vi "UART_Read_Write.vi"(0 "Transmit":refnum<k21>="Port8/DIO0", 5 "Receive":refnum<k21>="Port8/DIOCTL", 7 "baud rate (9600)":u32=9600, 9 "data bits (8)":i32=8 min=5 max=8 step=1, 11 "parity (0:none)":enum16{"None", "Odd", "Even", "Mark", "Space"}(ring), 12 "stop bits (10: 1 bit)":u16(ring)=10 items=["1.0"=10, "1.5"=15, "2.0"=20], 13 "Invert Polarity?":bool) -> ()   [LabVIEW 2011]
uses:
  <vilib>/rvi/eio/common/nirviEmuTemplateMethod_errors.vi
  <vilib>/rvi/interface/RandomDataEmulation/nirviRandomDataFPGAFIFO.vi
  <vilib>/rvi/interface/RandomDataEmulation/niFpgaRandomDataHandleErrors.vi
  Instance           1 27Saved   LV FPGA Serial Read .vi
  Instance           2 27Saved   LV FPGA Serial Read .vi
  Instance           3 27Saved   LV FPGA Serial Read .vi
  Instance           6 27Saved   LV FPGA Serial Read .vi
  <vilib>/eio/EIOMethodNode/EIOMethodNode.xnode
  <vilib>/rvi/DataTransferAndStorage/Container/XNode/niFpgaContainer.xnode
  <vilib>/rvi/interface/RandomDataEmulation/nirviRandomDataFpgaReadWriteTemplate.vi
  <vilib>/eio/EIONode/EIONode.xnode
panel:
  out "Read: Transmission Error":bool
  in  "stop":bool
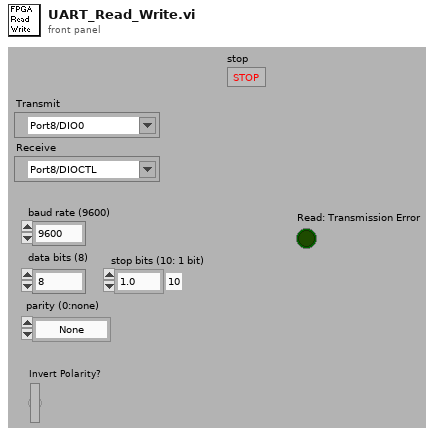
[diagram p1: front panel]
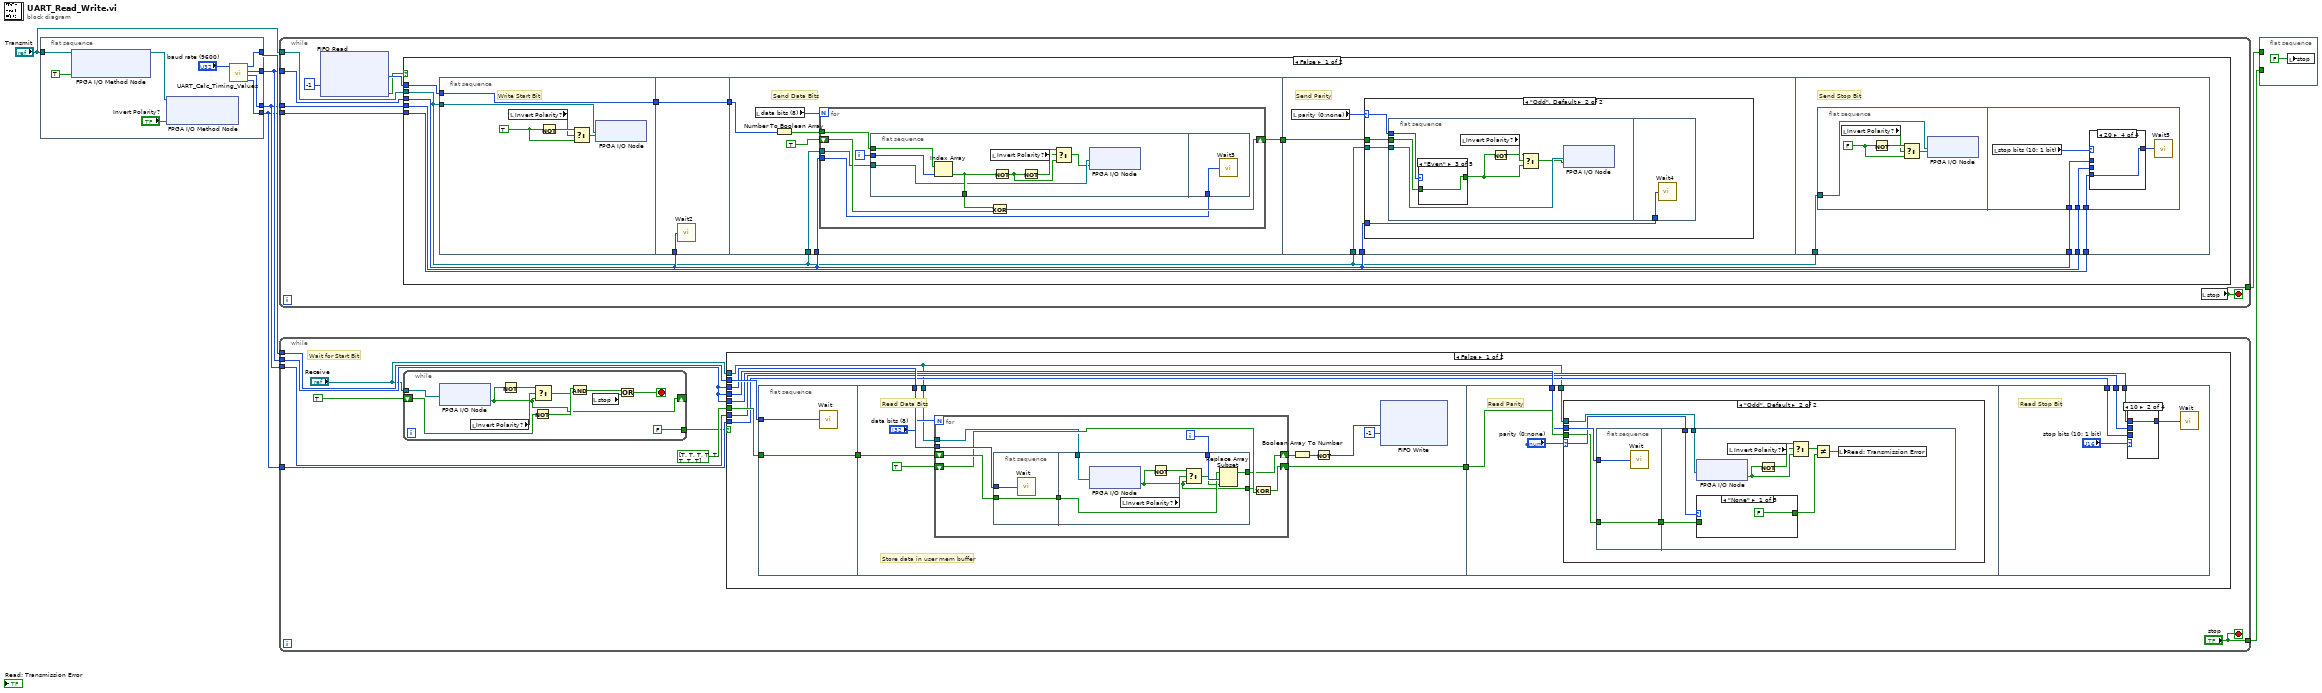
[diagram p0: block diagram]
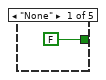
[diagram p3: hidden frame]
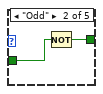
[diagram p4: hidden frame]
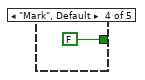
[diagram p5: hidden frame]
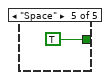
[diagram p6: hidden frame]
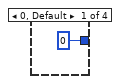
[diagram p7: hidden frame]
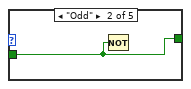
[diagram p12: hidden frame]
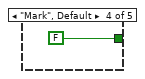
[diagram p14: hidden frame]
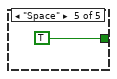
[diagram p15: hidden frame]
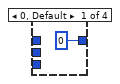
[diagram p16: hidden frame]
diagram:
  n1 = flat-sequence {
    tunnel: [w12] -> w6
    tunnel: [w15] -> w7
    tunnel: [w14] -> w5
    tunnel: [w13] -> w4
    tunnel: "Transmit" -> [w10]
    frame #0 {
      n2 = xnode "FPGA I/O Method Node"("FPGA I/O In"=w10, "Enable"=TRUE ("Digital Enable")) -> ("FPGA I/O Out"=w9:refnum<k21>)
      n3 = xnode "FPGA I/O Method Node"("FPGA I/O In"=w9, "Data"="Invert Polarity?") -> ()  [unwired: 1 out]
      n4 = call "UART_Calc_Timing_Values.vi"("baud rate (1000000)"="baud rate (9600)") -> ("Two Bit"=w13:u32, "One and Half Bit"=w14:u32, "One Bit"=w12:u32, "Half Bit"=w15:u32)  [unwired: 1 in, 2 out]
    }
  }
  n5 = while {
    tunnel: w4 -> [w24]
    tunnel: w5 -> [w23]
    tunnel: w6 -> [w22]
    tunnel: "Transmit" -> [w21]
    tunnel: [w17] -> w1
    stop <- w17 stop-if-true
    n6 = xnode ("FIFO Read")("Timeout"=-1) -> ("Element"=w20:u8, "Timed Out?"=w18:bool)  [unwired: 1 in, 1 out]
    n7 = case shown="False" w18 {
      tunnel: w24 -> [w29 _]
      tunnel: w23 -> [w28 _]
      tunnel: w22 -> [w27 _]
      tunnel: w21 -> [w26 _]
      tunnel: w20 -> [w25 _]
      frame False {
        n8 = flat-sequence {
          tunnel: w26 -> [w38]
          tunnel: w25 -> [w33]
          tunnel: [w33] -> w32
          tunnel: w27 -> [w40]
          tunnel: [w39] -> w31
          tunnel: w32 -> [w39]
          tunnel: w27 -> [w47]
          tunnel: [w45] -> w30
          tunnel: w26 -> [w42]
          tunnel: w31 -> [w41]
          tunnel: w27 -> [w66]
          tunnel: w30 -> [w67]
          tunnel: w26 -> [w64]
          tunnel: w27 -> [w89]
          tunnel: w28 -> [w88]
          tunnel: w29 -> [w87]
          tunnel: w26 -> [w86]
          frame #0 {
            w36 = TRUE
            # "Write Start Bit"
            n9 = local read "Invert Polarity?"() -> (w35:bool)
            n10 = Not(x=w36) -> (.not. x?=w37:bool)
            n11 = Select(t=w37, s=w35, f=w36) -> (s? t:f=w34:bool)
            n12 = xnode "FPGA I/O Node"("I/O Item"=w34, "FPGA I/O In"=w38) -> ()  [unwired: 1 out]
          }
          frame #1 {
            n13 = call "Wait2"("Count(Ticks)"=w40) -> ()  [unwired: 1 out]
          }
          frame #2 {
            # "Send Data Bits"
            n14 = local read "data bits (8)"() -> (w43:i32)
            n15 = Number To Boolean Array(number=w41) -> (Boolean array=w44:bool[])
            n16 = for {
              N: w43 -> [_]
              tunnel: w47 -> [w51]
              shift-right: [w54] -> w45
              shift-left: TRUE -> [w53]
              tunnel: w44 -> [w50]
              tunnel: w42 -> [w48]
              i -> [w52]
              n17 = flat-sequence {
                tunnel: w52 -> [w62]
                tunnel: w50 -> [w61]
                tunnel: [w60] -> w49
                tunnel: w48 -> [w59]
                tunnel: w51 -> [w63]
                frame #0 {
                  n18 = Index Array(array=w61, index=w62) -> (element=w60:bool)
                  n19 = local read "Invert Polarity?"() -> (w56:bool)
                  n20 = Not(x=w60) -> (.not. x?=w57:bool)
                  n21 = Not(x=w57) -> (.not. x?=w58:bool)
                  n22 = Select(t=w58, s=w56, f=w57) -> (s? t:f=w55:bool)
                  n23 = xnode "FPGA I/O Node"("I/O Item"=w55, "FPGA I/O In"=w59) -> ()  [unwired: 1 out]
                }
                frame #1 {
                  n24 = call "Wait3"("Count(Ticks)"=w63) -> ()  [unwired: 1 out]
                }
              }
              n25 = Exclusive Or(1:w53, 2:w49) -> (0:w54:bool)
            }
          }
          frame #3 {
            # "Send Parity"
            n26 = local read "parity (0:none)"() -> (w65:enum16{"None", "Odd", "Even", "Mark", "Space"})
            n27 = case shown="\"Odd\", Default" w65 {
              selector: w65 -> [_ w71]
              tunnel: w67 -> [_ w70]
              tunnel: w66 -> [_ w69]
              tunnel: w64 -> [_ w68]
              frame "None" {
              }
              frame "Odd", Default {
                n28 = flat-sequence {
                  tunnel: w70 -> [w77]
                  tunnel: w71 -> [w78]
                  tunnel: w68 -> [w76]
                  tunnel: w69 -> [w85]
                  frame #0 {
                    n29 = case shown="\"Even\"" w78 {
                      tunnel: w77 -> [_ w81 w82 _ _]
                      tunnel: [FALSE ("y") w80 w82 FALSE ("y") TRUE ("y")] -> w73
                      frame "None" {
                      }
                      frame "Odd" {
                        n30 = Not(x=w81) -> (.not. x?=w80:bool)
                      }
                      frame "Even" {
                      }
                      frame "Mark", Default {
                      }
                      frame "Space" {
                      }
                    }
                    n31 = local read "Invert Polarity?"() -> (w75:bool)
                    n32 = Not(x=w73) -> (.not. x?=w74:bool)
                    n33 = Select(t=w74, s=w75, f=w73) -> (s? t:f=w72:bool)
                    n34 = xnode "FPGA I/O Node"("I/O Item"=w72, "FPGA I/O In"=w76) -> ()  [unwired: 1 out]
                  }
                  frame #1 {
                    n35 = call "Wait4"("Count(Ticks)"=w85) -> ()  [unwired: 1 out]
                  }
                }
              }
            }
          }
          frame #4 {
            # "Send Stop Bit"
            n36 = flat-sequence {
              tunnel: w86 -> [w94]
              tunnel: w89 -> [w99]
              tunnel: w88 -> [w98]
              tunnel: w87 -> [w97]
              frame #0 {
                w92 = FALSE
                n37 = local read "Invert Polarity?"() -> (w91:bool)
                n38 = Not(x=w92) -> (.not. x?=w93:bool)
                n39 = Select(t=w93, s=w91, f=w92) -> (s? t:f=w90:bool)
                n40 = xnode "FPGA I/O Node"("I/O Item"=w90, "FPGA I/O In"=w94) -> ()  [unwired: 1 out]
              }
              frame #1 {
                n41 = local read "stop bits (10: 1 bit)"() -> (w95:u16)
                n42 = case shown="20" w95 {
                  tunnel: w99 -> [_ w101 _ _]
                  tunnel: w98 -> [_ _ w102 _]
                  tunnel: w97 -> [_ _ _ w103]
                  tunnel: [u32 0 ("One Bit") w101 w102 w103] -> w96
                  frame 0, Default {
                  }
                  frame 10 {
                  }
                  frame 15 {
                  }
                  frame 20 {
                  }
                }
                n43 = call "Wait5"("Count(Ticks)"=w96) -> ()  [unwired: 1 out]
              }
            }
          }
        }
      }
      frame True {
      }
    }
    n44 = local read "stop"() -> (w17:bool)
  }
  n45 = while {
    tunnel: w4 -> [w111]
    tunnel: w5 -> [w110]
    tunnel: w6 -> [w109]
    tunnel: w7 -> [w108]
    tunnel: ["stop"] -> w2
    stop <- "stop" stop-if-true
    # "Wait for Start Bit"
    n46 = while {
      tunnel: [FALSE] -> w107
      shift-right: [w113] -> _
      shift-left: TRUE -> [w122]
      tunnel: "Receive" -> [w117]
      stop <- w118 stop-if-true
      n47 = xnode "FPGA I/O Node"("FPGA I/O In"=w117) -> ("I/O Item"=w113:bool)  [unwired: 1 out]
      n48 = local read "Invert Polarity?"() -> (w115:bool)
      n49 = Not(x=w113) -> (.not. x?=w116:bool)
      n50 = Not(x=w122) -> (.not. x?=w121:bool)
      n51 = Select(t=w116, s=w115, f=w113) -> (s? t:f=w114:bool)
      n52 = And(x=w121, y=w114) -> (x .and. y?=w119:bool)
      n53 = local read "stop"() -> (w120:bool)
      n54 = Or(x=w119, y=w120) -> (x .or. y?=w118:bool)
    }
    n55 = case shown="False" w107 {
      tunnel: bool[] [TRUE, TRUE, TRUE, TRUE, TRUE, TRUE, TRUE, TRUE] -> [w132 _]
      tunnel: w108 -> [w131 _]
      tunnel: w109 -> [w130 _]
      tunnel: w109 -> [w129 _]
      tunnel: w109 -> [w128 _]
      tunnel: w110 -> [w127 _]
      tunnel: w111 -> [w126 _]
      tunnel: "Receive" -> [w124 _]
      frame False {
        n56 = flat-sequence {
          tunnel: [w135] -> w133
          tunnel: w132 -> [w135]
          tunnel: w131 -> [w134]
          tunnel: w133 -> [w145]
          tunnel: w130 -> [w144]
          tunnel: [w140] -> w125
          tunnel: w124 -> [w138]
          tunnel: w129 -> [w166]
          tunnel: w125 -> [w168]
          tunnel: w124 -> [w165]
          tunnel: w128 -> [w193]
          tunnel: w127 -> [w192]
          tunnel: w126 -> [w191]
          frame #0 {
            n57 = call "Wait"("Count(Ticks)"=w134) -> ()  [unwired: 1 out]
          }
          frame #1 {
            # "Store data in user mem buffer"
            # "Read Data Bits"
            n58 = for {
              N: "data bits (8)" -> [_]
              shift-right: [w148] -> w143
              shift-left: w145 -> [w154]
              tunnel: w144 -> [w152]
              shift-right: [w151] -> w140
              shift-left: TRUE -> [w150]
              tunnel: w138 -> [w146]
              i -> [w147]
              n59 = flat-sequence {
                tunnel: w154 -> [w156]
                tunnel: [w156] -> w153
                tunnel: w152 -> [w155]
                tunnel: w147 -> [w164]
                tunnel: w153 -> [w163]
                tunnel: [w162] -> w148
                tunnel: [w157] -> w149
                tunnel: w146 -> [w161]
                frame #0 {
                  n60 = call "Wait"("Count(Ticks)"=w155) -> ()  [unwired: 1 out]
                }
                frame #1 {
                  n61 = xnode "FPGA I/O Node"("FPGA I/O In"=w161) -> ("I/O Item"=w157:bool)  [unwired: 1 out]
                  n62 = local read "Invert Polarity?"() -> (w160:bool)
                  n63 = Not(x=w157) -> (.not. x?=w159:bool)
                  n64 = Select(t=w159, s=w160, f=w157) -> (s? t:f=w158:bool)
                  n65 = Replace Array Subset(array=w163, new element=w158, index=w164) -> (w162:bool[])
                }
              }
              n66 = Exclusive Or(1:w150, 2:w149) -> (0:w151:bool)
            }
            n67 = Boolean Array To Number(Boolean array=w143) -> (number=w142:u8)
            n68 = Not(x=w142) -> (.not. x?=w137:u8)
            n69 = xnode ("FIFO Write")("Element"=w137, "Timeout"=-1) -> ()  [unwired: 1 in, 2 out]
          }
          frame #2 {
            # "Read Parity"
            n70 = case shown="\"Odd\", Default" "parity (0:none)" {
              selector: "parity (0:none)" -> [_ w172]
              tunnel: w168 -> [_ w170]
              tunnel: w166 -> [_ w173]
              tunnel: w165 -> [_ w169]
              frame "None" {
              }
              frame "Odd", Default {
                n71 = flat-sequence {
                  tunnel: w173 -> [w175]
                  tunnel: [w174] -> w171
                  tunnel: w170 -> [w174]
                  tunnel: w172 -> [w184]
                  tunnel: w171 -> [w182]
                  tunnel: w169 -> [w180]
                  frame #0 {
                    n72 = call "Wait"("Count(Ticks)"=w175) -> ()  [unwired: 1 out]
                  }
                  frame #1 {
                    n73 = xnode "FPGA I/O Node"("FPGA I/O In"=w180) -> ("I/O Item"=w177:bool)  [unwired: 1 out]
                    n74 = case shown="\"None\"" w184 {
                      tunnel: w182 -> [_ w186 w187 _ _]
                      tunnel: [FALSE ("y") w186 w187 FALSE ("y") TRUE ("y")] -> w183
                      frame "None" {
                      }
                      frame "Odd" {
                        n75 = Not(x=w186) -> ()  [unwired: 1 out]
                      }
                      frame "Even" {
                      }
                      frame "Mark", Default {
                      }
                      frame "Space" {
                      }
                    }
                    n76 = local read "Invert Polarity?"() -> (w178:bool)
                    n77 = Not(x=w177) -> (.not. x?=w179:bool)
                    n78 = Select(t=w179, s=w178, f=w177) -> (s? t:f=w176:bool)
                    n79 = Not Equal?(x=w176, y=w183) -> (x != y?=w181:bool)
                    n80 = local write "Read: Transmission Error"(w181) -> ()
                  }
                }
              }
            }
          }
          frame #3 {
            # "Read Stop Bit"
            n81 = case shown="10" "stop bits (10: 1 bit)" {
              tunnel: w193 -> [_ w196 _ _]
              tunnel: w192 -> [_ _ w197 _]
              tunnel: w191 -> [_ _ _ w198]
              tunnel: [u32 0 ("One Bit") w196 w197 w198] -> w190
              frame 0, Default {
              }
              frame 10 {
              }
              frame 15 {
              }
              frame 20 {
              }
            }
            n82 = call "Wait"("Count(Ticks)"=w190) -> ()  [unwired: 1 out]
          }
        }
      }
      frame True {
      }
    }
  }
  n83 = flat-sequence {
    tunnel: w2 -> [_]
    tunnel: w1 -> [_]
    frame #0 {
      n84 = local write "stop"(FALSE ("stop")) -> ()
    }
  }
